vi "Begin.vi"(8 "error in":errorcluster) -> (0 "error out":errorcluster)   [LabVIEW 2017]
doc: "Called before other user functions, this VI is expected to open initial I/O refnums, load in file data, and do all program initialization. Notice that the <B>error out</B> terminal is simply used for data flow. Wiring it to other structures or subVIs ensures that this VI runs first."
uses:
  <vilib>/Rock Robotics/WPI/Joystick/WPI_JoystickDeviceEnum.ctl
  <vilib>/Rock Robotics/SystemInterfaces/AI/FPGA_AIChannel.ctl
  <vilib>/Rock Robotics/WPI/ThirdParty/Phoenix-LabVIEW/Motor Controller/Controls/CTRE_Phoenix_MotorControl_ControlMode.ctl
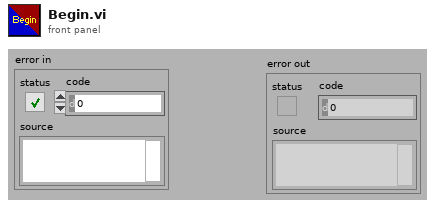
[diagram p1: front panel]
types:
  T1 = typedef "CTRE_Phoenix_MotorControl_ControlMode.ctl" = u16
  T2 = typedef "FPGA_AIChannel.ctl" = enum8{"AI 0", "AI 1", "AI 2", "AI 3", "AI MXP 0", "AI MXP 1", "AI MXP 2", "AI MXP 3", "Invalid"}
  T3 = typedef "WPI_JoystickDeviceEnum.ctl" = enum16{"USB 0", "USB 1", "USB 2", "USB 3", "USB 4", "USB 5"}
  T4 = typedef "WPI_MotorControlDeviceRef.ctl" = cluster{"DeviceStatus":errorcluster, "Type":T5, "PWM":cluster{"PWM Channel":T6, "DeadBand":T7}, "CAN":cluster{"Device Number":u8, "SetOutput VI Ref":variant, "GetOutput VI Ref":variant, "Enable VI Ref":variant, "Disable VI Ref":variant, "Data":variant}, "Invert":bool, "DIO PWM":cluster{"PWM \"Enable\" Channel":T6, "DIOChannel":T8, "PWM Rate":dbl}}
  T5 = typedef "WPI_MotorControlType.ctl" = enum16{"PWM", "CAN", "DIO PWM"}
  T6 = typedef "FPGA_DIOPWMChannel.ctl" = enum8{"PWM 0", "PWM 1", "PWM 2", "PWM 3", "PWM 4", "PWM 5", "PWM 6", "PWM 7", "PWM 8", "PWM 9", "PWM MXP 0", "PWM MXP 1", "PWM MXP 2", "PWM MXP 3", "PWM MXP 4", "PWM MXP 5", "PWM MXP 6", "PWM MXP 7", "PWM MXP 8", "PWM MXP 9", "Invalid"}
  T7 = typedef "WPI_PWMDeadband.ctl" = cluster{"Name":string, "maxPositivePwm":i32, "minPositivePwm":i32, "centerPwm":i32, "maxNegativePwm":i32, "minNegativePwm":i32, "angularRange":u16}
  T8 = typedef "FPGA_DIOChannel.ctl" = enum8{"DIO 0", "DIO 1", "DIO 2", "DIO 3", "DIO 4", "DIO 5", "DIO 6", "DIO 7", "DIO 8", "DIO 9", "DIO MXP 0", "DIO MXP 1", "DIO MXP 2", "DIO MXP 3", "DIO MXP 4", "DIO MXP 5", "DIO MXP 6", "DIO MXP 7", "DIO MXP 8", "DIO MXP 9", "DIO MXP 10", "DIO MXP 11", "DIO MXP 12", "DIO MXP 13", "DIO MXP 14", "DIO MXP 15", "SPI Port CS1", "SPI Port CS2", "SPI Port CS3", "SPI Port MISO", "SPI Port MOSI", "Invalid"}
  T9 = typedef "WPI_JoystickDevRef.ctl" = cluster{"Device":T3}
  T10 = typedef "WPI_AnalogChannelDevRef.ctl" = cluster{"DevStatus":errorcluster, "Analog Channel":T2}
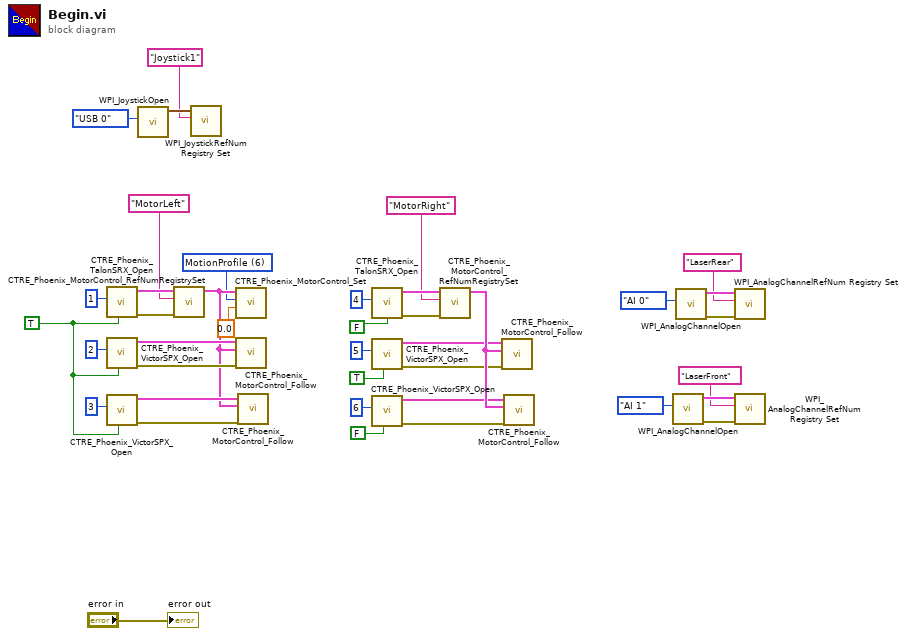
[diagram p0: block diagram]
diagram:
  w2 = T1 6 items=["PercentOutput"=0, "Position"=1, "Velocity"=2, "Current"=3, "Follower"=5, "MotionProfile"=6, "MotionMagic"=7, "MotionMagicArc"=8, "MotionProfileArc"=10, "Disabled"=15] ("Control Mode")
  w15 = TRUE
  n1 = call <vilib>:"CTRE_Phoenix_TalonSRX_Open.vi"("Invert"=w15, "Device Number"=u8 1) -> ("error out"=w39:errorcluster, "CAN Talon SRX Ref"=w38:T4)  [unwired: 8 in]
  n2 = call <vilib>:"CTRE_Phoenix_VictorSPX_Open.vi"("Invert"=w15, "Device Number"=u8 2) -> ("error out"=w36:errorcluster, "CAN Talon SRX Ref"=w37:T4)  [unwired: 8 in]
  n3 = call <vilib>:"CTRE_Phoenix_VictorSPX_Open.vi"("Invert"=w15, "Device Number"=u8 3) -> ("error out"=w34:errorcluster, "CAN Talon SRX Ref"=w35:T4)  [unwired: 8 in]
  n4 = call <vilib>:"WPI_JoystickOpen.vi"("JoystickDevice"=WPI_JoystickDeviceEnum."USB 0") -> ("JoystickDevRef"=w18:T9)  [unwired: 10 in]
  n5 = call <vilib>:"CTRE_Phoenix_MotorControl_RefNumRegistrySet.vi"("error in (no error)"=w39, "refnum name"="MotorLeft", "PhoenixMotorControlDevRef"=w38) -> ("PhoenixMotorControlDevRef"=w3:T4)  [unwired: 7 in, 1 out]
  n6 = call <vilib>:"WPI_JoystickRefNum Registry Set.vi"("refnum name"="Joystick1", "JoystickDevRef"=w18) -> ()  [unwired: 8 in, 2 out]
  n7 = call <vilib>:"CTRE_Phoenix_MotorControl_Set.vi"("Output"=0.0, "Control Mode"=w2, "PhoenixMotorControlDevRef"=w3) -> ()  [unwired: 7 in, 2 out]
  n8 = call <vilib>:"CTRE_Phoenix_MotorControl_Follow.vi"("error in (no error)"=w36, "Master Controller to Follow"=w3, "PhoenixMotorControlDevRef"=w37) -> ()  [unwired: 7 in, 2 out]
  n9 = call <vilib>:"CTRE_Phoenix_MotorControl_Follow.vi"("error in (no error)"=w34, "Master Controller to Follow"=w3, "PhoenixMotorControlDevRef"=w35) -> ()  [unwired: 7 in, 2 out]
  n10 = call <vilib>:"CTRE_Phoenix_TalonSRX_Open.vi"("Invert"=FALSE, "Device Number"=u8 4) -> ("error out"=w33:errorcluster, "CAN Talon SRX Ref"=w32:T4)  [unwired: 8 in]
  n11 = call <vilib>:"CTRE_Phoenix_VictorSPX_Open.vi"("Invert"=TRUE, "Device Number"=u8 5) -> ("error out"=w29:errorcluster, "CAN Talon SRX Ref"=w30:T4)  [unwired: 8 in]
  n12 = call <vilib>:"CTRE_Phoenix_VictorSPX_Open.vi"("Invert"=FALSE, "Device Number"=u8 6) -> ("error out"=w27:errorcluster, "CAN Talon SRX Ref"=w28:T4)  [unwired: 8 in]
  n13 = call <vilib>:"CTRE_Phoenix_MotorControl_RefNumRegistrySet.vi"("error in (no error)"=w33, "refnum name"="MotorRight", "PhoenixMotorControlDevRef"=w32) -> ("PhoenixMotorControlDevRef"=w31:T4)  [unwired: 7 in, 1 out]
  n14 = call <vilib>:"CTRE_Phoenix_MotorControl_Follow.vi"("error in (no error)"=w29, "Master Controller to Follow"=w31, "PhoenixMotorControlDevRef"=w30) -> ()  [unwired: 7 in, 2 out]
  n15 = call <vilib>:"CTRE_Phoenix_MotorControl_Follow.vi"("error in (no error)"=w27, "Master Controller to Follow"=w31, "PhoenixMotorControlDevRef"=w28) -> ()  [unwired: 7 in, 2 out]
  n16 = call <vilib>:"WPI_AnalogChannelOpen.vi"("Analog Channel"=FPGA_AIChannel."AI 1") -> ("error out"=w12:errorcluster, "AIDeviceRef"=w11:T10)  [unwired: 9 in]
  n17 = call <vilib>:"WPI_AnalogChannelOpen.vi"("Analog Channel"=FPGA_AIChannel."AI 0") -> ("error out"=w14:errorcluster, "AIDeviceRef"=w13:T10)  [unwired: 9 in]
  n18 = call <vilib>:"WPI_AnalogChannelRefNum Registry Set.vi"("error in (no error)"=w14, "refnum name"="LaserRear", "AIDeviceRef"=w13) -> ()  [unwired: 7 in, 2 out]
  n19 = call <vilib>:"WPI_AnalogChannelRefNum Registry Set.vi"("error in (no error)"=w12, "refnum name"="LaserFront", "AIDeviceRef"=w11) -> ()  [unwired: 7 in, 2 out]
  "error out" <- "error in"
